vi "TP_IsFinished.vi"(8 "error in (no error)":errorcluster, 10 "t":dbl=-1.0, 11 "TrapezoidalProfile in":refnum<class "TrapezoidalProfile.lvclass">) -> (0 "error out":errorcluster, 2 "Is Finished?":bool, 3 "TrapezoidalProfile out":refnum<class "TrapezoidalProfile.lvclass">)   [LabVIEW 2018, in "TrapezoidalProfile.lvclass"]
uses:
  TrapezoidalProfile.lvclass
  TrapezoidalProfile.lvclass/TrapezoidalProfile.ctl
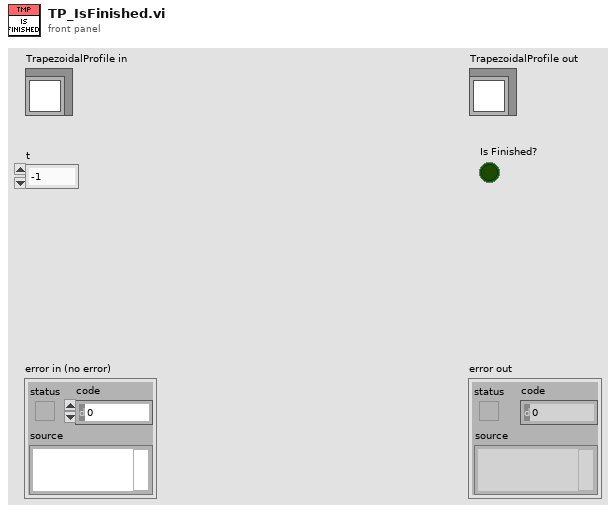
[diagram p1: front panel]
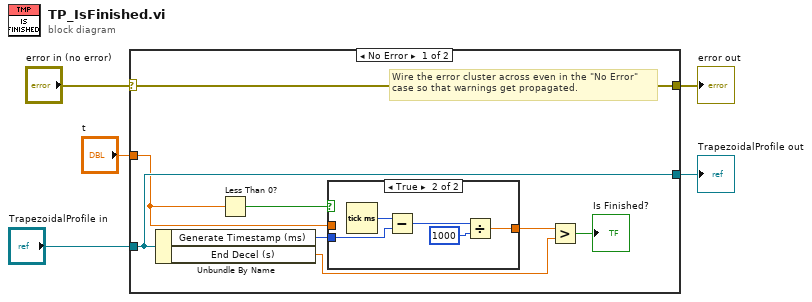
[diagram p0: block diagram]
diagram:
  n1 = case shown="No Error" "error in (no error)" {
    selector: "error in (no error)" -> [w13 w21]
    tunnel: [w13 w21] -> w4
    tunnel: [w12 w20] -> w2
    tunnel: "TrapezoidalProfile in" -> [w12 w20]
    tunnel: "t" -> [w6 _]
    frame No Error {
      # "Wire the error cluster across even in the \"No Error\"\ncase so that warnings get propagated."
      n2 = Unbundle By Name(w12) -> ("Generate Timestamp (ms)"=w9:u32, "End Decel (s)"=w10:dbl)
      n3 = Less Than 0?(x=w6) -> (x < 0?=w7:bool)
      n4 = case shown="True" w7 {
        tunnel: w9 -> [_ w19]
        tunnel: [w14 w15] -> w8
        tunnel: w6 -> [w14 _]
        frame False {
        }
        frame True {
          n5 = Tick Count (ms)() -> (millisecond timer value=w18:u32)
          n6 = Subtract(x=w18, y=w19) -> (x-y=w17:u32)
          n7 = Divide(x=w17, y=u32 1000) -> (x/y=w15:dbl)
        }
      }
      n8 = Greater?(x=w8, y=w10) -> (0:→"Is Finished?":bool)
    }
    frame Error {
    }
  }
  "error out" <- w4
  "TrapezoidalProfile out" <- w2
